vi "Terminate Application.vi"(8 "error in (no error)":errorcluster, 11 "Application in":refnum<vi>) -> ()   [LabVIEW 2017]
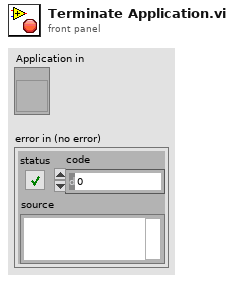
[diagram p1: front panel]
types:
  T1 = enum32{"invalid app kind", "Development System", "Run Time System", "Student Edition", "Embedded LabVIEW", "Evaluation", "Custom"}
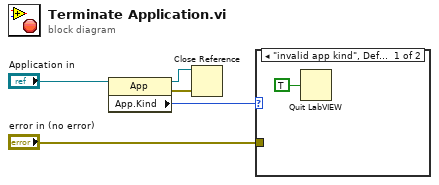
[diagram p0: block diagram]
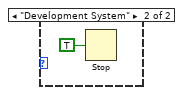
[diagram p2: hidden frame]
diagram:
  n1 = property class="App"(reference="Application in") -> (reference out=w5:refnum<vi>, error out=w4:errorcluster, "App.Kind"=w3:T1)  [unwired: 1 in]
  n2 = Close Reference(reference=w5, error in (no error)=w4) -> ()  [unwired: 1 out]
  n3 = case shown="\"invalid app kind\", Default" w3 {
    tunnel: "error in (no error)" -> [_ _]
    frame "invalid app kind", Default {
      n4 = Quit LabVIEW(quit? (T)=TRUE) -> ()
    }
    frame "Development System" {
      n5 = Stop(stop? (T)=TRUE) -> ()
    }
  }
